vi "Image_Create_Testpattern.vi"(7 "Pattern":enum16{"24 Color Checker", "Customized Pure"}(ring), 8 "error in (no error)":errorcluster, 9 "Pure Color Pattern Parameters":cluster{"R":u8, "G":u8, "B":u8}={"R"=255, "G"=255, "B"=255}, 10 "Image Configuration":T1={"Width"=1920, "Height"=1080}) -> (0 "error out":errorcluster, 1 "Image":T2(plugin-control), 2 "Image Configuration Out":T1={"Width"=1920, "Height"=1080}, 3 "RGB U8":u8[](array[numeric]))   [LabVIEW 2020]
uses:
  ctl/Image_Configuration.ctl
  <vilib>/vision/Image Controls.llb/IMAQ Image.ctl
  <vilib>/vision/NI_Vision_Development_Module.lvlib
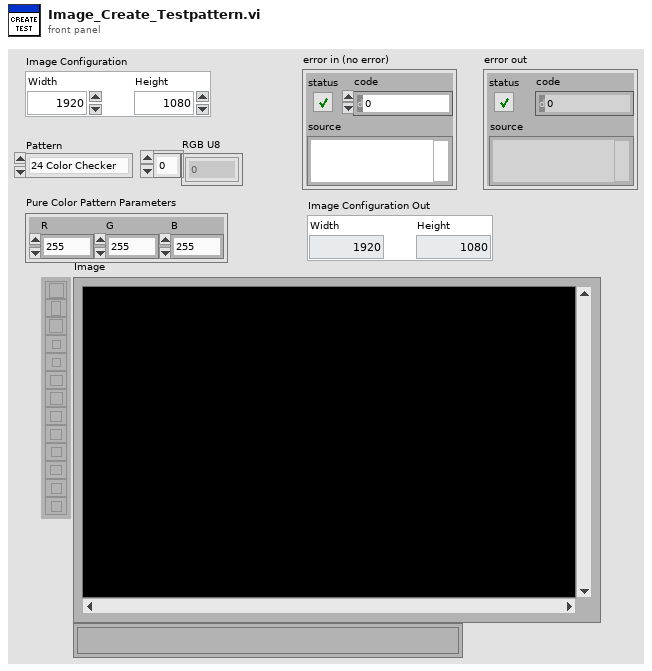
[diagram p1: front panel]
types:
  T1 = typedef "Image_Configuration.ctl" = cluster{"Width":i32, "Height":i32}
  T2 = typedef "IMAQ Image.ctl" = refnum<image>
  T3 = typedef "Image Type" = u32
  T4 = cluster{"Red (or Hue) value":u8, "Green (or Sat) value":u8, "Blue (or Light or Val) value":u8}[]
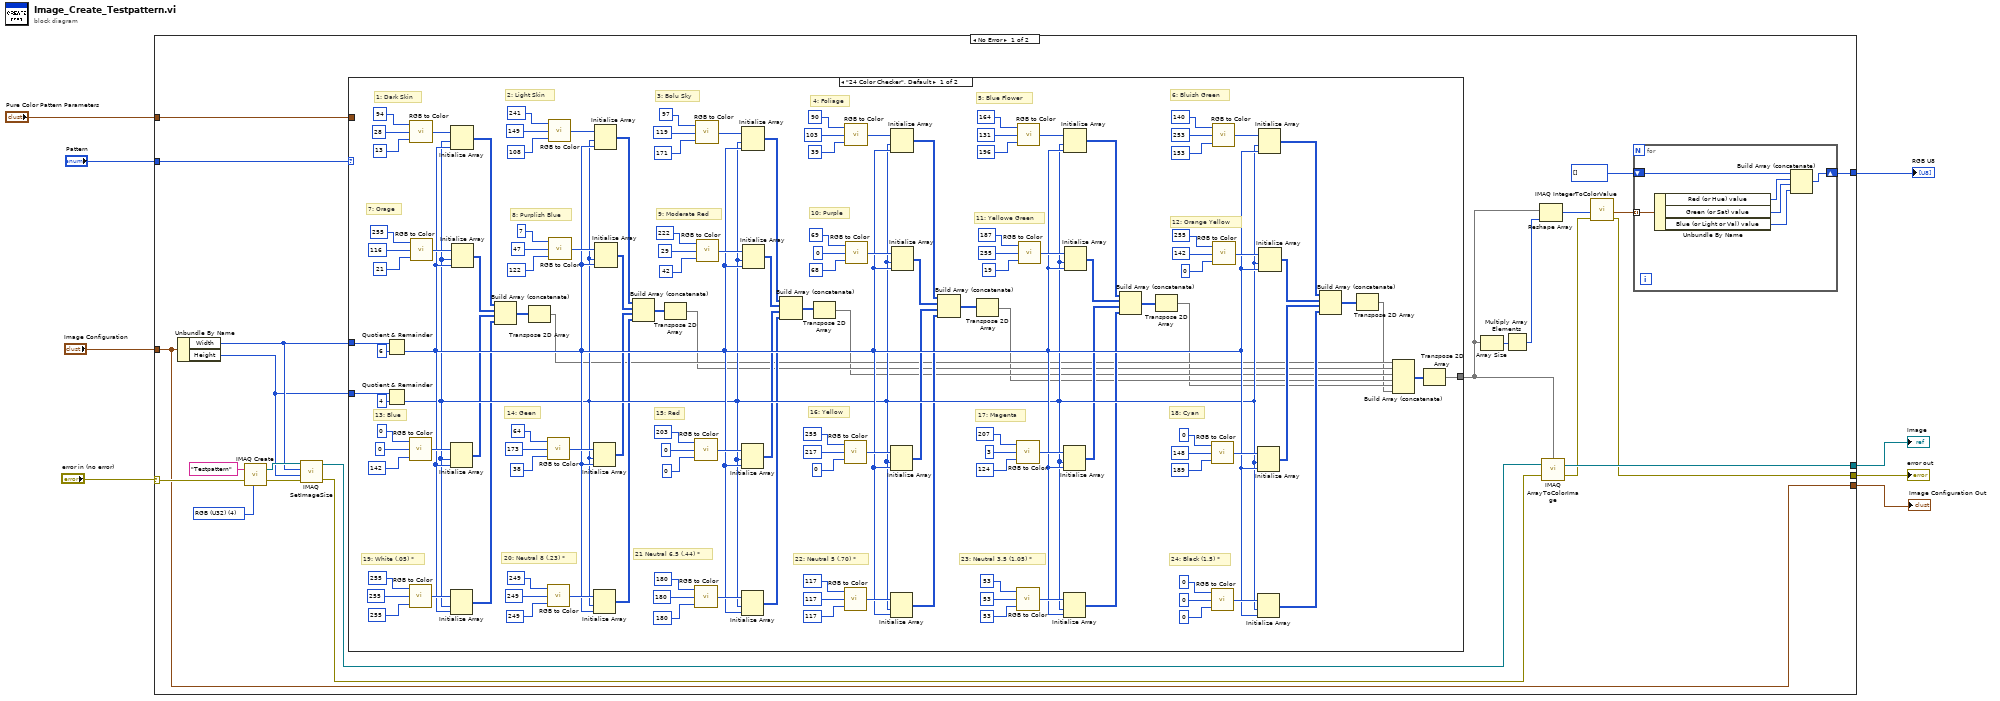
[diagram p0: block diagram]
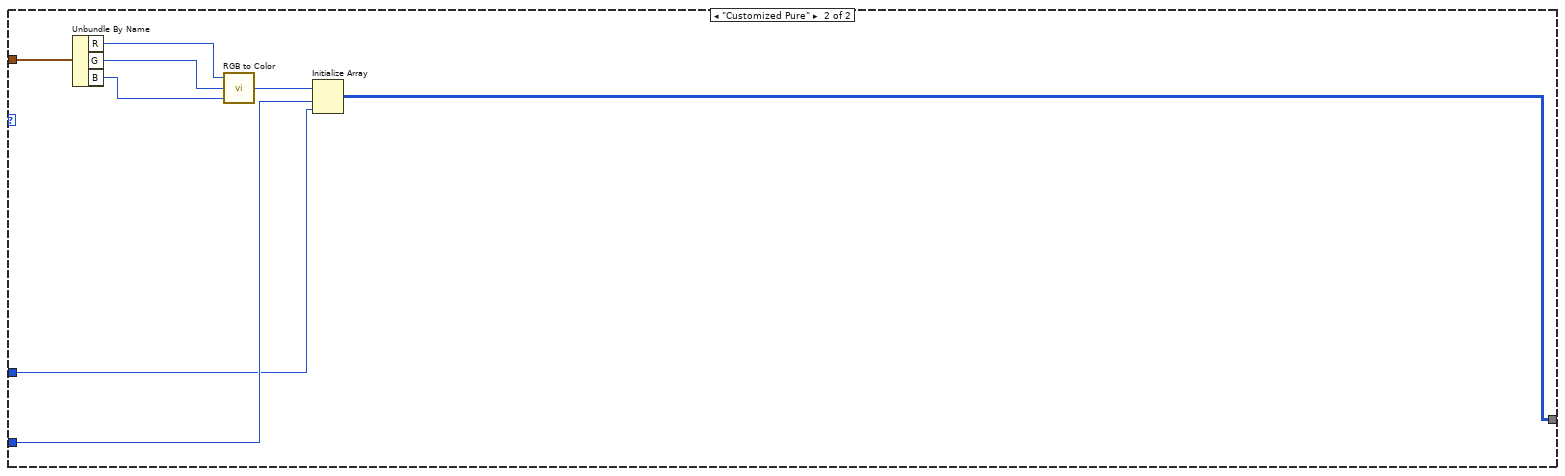
[diagram p2: hidden frame]
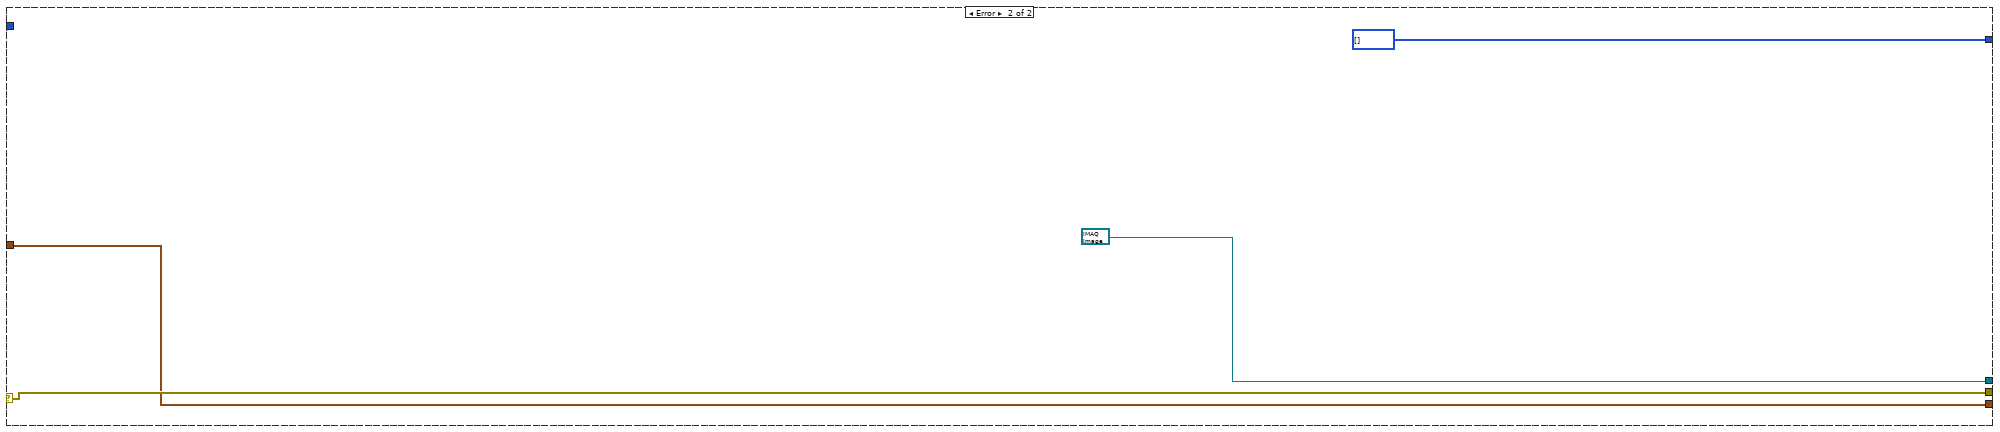
[diagram p3: hidden frame]
diagram:
  n1 = case shown="No Error" "error in (no error)" {
    selector: "error in (no error)" -> [w27 w187]
    tunnel: "Image Configuration" -> [w10 w185]
    tunnel: [w23 T2 refnum ("Image Out")] -> w6
    tunnel: [w14 w187] -> w5
    tunnel: [w15 u8[] []] -> w4
    tunnel: "Pattern" -> [w13 _]
    tunnel: [w10 w185] -> w2
    tunnel: "Pure Color Pattern Parameters" -> [w9 _]
    frame No Error {
      w30 = T3 4 items=["Grayscale (U8)", "Grayscale (I16)", "Grayscale (SGL)", "Complex (CSG)", "RGB (U32)", "HSL (U32)", "RGB (U64)", "Grayscale (U16)"] ("Image Type")
      n2 = Unbundle By Name(w10) -> ("Width"=w25:i32, "Height"=w24:i32)
      n3 = call "IMAQ Create"("Image Name"="Testpattern", "Image Type"=w30, "error in (no error)"=w27) -> ("New Image"=w28:T2, "error out"=w29:errorcluster)  [unwired: 2 in]
      n4 = call "IMAQ SetImageSize"("error in (no error)"=w29, "Y Resolution"=w24, "X Resolution"=w25, "Image"=w28) -> ("error out"=w11:errorcluster, "Image Out"=w12:T2)  [unwired: 1 in]
      n5 = case shown="\"24 Color Checker\", Default" w13 {
        tunnel: w25 -> [w167 w172]
        tunnel: w24 -> [w165 w173]
        tunnel: [w31 w171] -> w20
        tunnel: w9 -> [_ w177]
        frame "24 Color Checker", Default {
          # "24: Black (1.5) *"
          # "23: Neutral 3.5 (1.05) *"
          # "22: Neutral 5 (.70) *"
          # "21 Neutral 6.5 (.44) *"
          # "20: Neutral 8 (.23) *"
          # "19: White (.05) *"
          # "18: Cyan"
          # "17: Magenta"
          # "16: Yellow"
          # "15: Red"
          # "14: Geen"
          # "13: Blue"
          # "12: Orange Yellow"
          # "11: Yellowe Green"
          # "10: Purple"
          # "9: Moderate Red"
          # "8: Purplish Blue"
          # "7: Orage"
          # "6: Bluish Green"
          # "5: Blue Flower"
          # "4: Foliage"
          # "3: Bolu Sky"
          # "2: Light Skin"
          # "1: Dark Skin"
          n6 = Quotient & Remainder(x=w167, y=6) -> (floor(x/y)=w70:i32)  [unwired: 1 out]
          n7 = Quotient & Remainder(x=w165, y=4) -> (floor(x/y)=w69:i32)  [unwired: 1 out]
          n8 = call <vilib>:"RGB to Color.vi"("B"=u8 142, "G"=u8 0, "R"=u8 0) -> ("Color"=w116:u32)
          n9 = call <vilib>:"RGB to Color.vi"("B"=u8 255, "G"=u8 255, "R"=u8 255) -> ("Color"=w92:u32)
          n10 = call <vilib>:"RGB to Color.vi"("B"=u8 13, "G"=u8 28, "R"=u8 94) -> ("Color"=w168:u32)
          n11 = call <vilib>:"RGB to Color.vi"("B"=u8 21, "G"=u8 116, "R"=u8 255) -> ("Color"=w140:u32)
          n12 = Initialize Array(w116, w69, w70) -> (w66:u32[][])
          n13 = Initialize Array(w92, w69, w70) -> (w65:u32[][])
          n14 = Initialize Array(w168, w69, w70) -> (w68:u32[][])
          n15 = Initialize Array(w140, w69, w70) -> (w67:u32[][])
          n16 = Build Array (concatenate)(w68, w67, w66, w65) -> (w44:u32[][])
          n17 = Transpose 2D Array(2D array=w44) -> (transposed array=w38:u32[][])
          n18 = call <vilib>:"RGB to Color.vi"("B"=u8 38, "G"=u8 173, "R"=u8 64) -> ("Color"=w112:u32)
          n19 = call <vilib>:"RGB to Color.vi"("B"=u8 249, "G"=u8 249, "R"=u8 249) -> ("Color"=w88:u32)
          n20 = call <vilib>:"RGB to Color.vi"("B"=u8 108, "G"=u8 149, "R"=u8 241) -> ("Color"=w160:u32)
          n21 = call <vilib>:"RGB to Color.vi"("B"=u8 122, "G"=u8 47, "R"=u8 7) -> ("Color"=w136:u32)
          n22 = Initialize Array(w112, w69, w70) -> (w62:u32[][])
          n23 = Initialize Array(w88, w69, w70) -> (w61:u32[][])
          n24 = Initialize Array(w160, w69, w70) -> (w64:u32[][])
          n25 = Initialize Array(w136, w69, w70) -> (w63:u32[][])
          n26 = Build Array (concatenate)(w64, w63, w62, w61) -> (w43:u32[][])
          n27 = Transpose 2D Array(2D array=w43) -> (transposed array=w37:u32[][])
          n28 = call <vilib>:"RGB to Color.vi"("B"=u8 0, "G"=u8 0, "R"=u8 203) -> ("Color"=w108:u32)
          n29 = call <vilib>:"RGB to Color.vi"("B"=u8 180, "G"=u8 180, "R"=u8 180) -> ("Color"=w84:u32)
          n30 = call <vilib>:"RGB to Color.vi"("B"=u8 171, "G"=u8 119, "R"=u8 97) -> ("Color"=w156:u32)
          n31 = call <vilib>:"RGB to Color.vi"("B"=u8 42, "G"=u8 29, "R"=u8 222) -> ("Color"=w132:u32)
          n32 = Initialize Array(w108, w69, w70) -> (w58:u32[][])
          n33 = Initialize Array(w84, w69, w70) -> (w57:u32[][])
          n34 = Initialize Array(w156, w69, w70) -> (w60:u32[][])
          n35 = Initialize Array(w132, w69, w70) -> (w59:u32[][])
          n36 = Build Array (concatenate)(w60, w59, w58, w57) -> (w42:u32[][])
          n37 = Transpose 2D Array(2D array=w42) -> (transposed array=w36:u32[][])
          n38 = call <vilib>:"RGB to Color.vi"("B"=u8 0, "G"=u8 217, "R"=u8 255) -> ("Color"=w107:u32)
          n39 = call <vilib>:"RGB to Color.vi"("B"=u8 117, "G"=u8 117, "R"=u8 117) -> ("Color"=w83:u32)
          n40 = call <vilib>:"RGB to Color.vi"("B"=u8 39, "G"=u8 103, "R"=u8 90) -> ("Color"=w155:u32)
          n41 = call <vilib>:"RGB to Color.vi"("B"=u8 68, "G"=u8 0, "R"=u8 69) -> ("Color"=w131:u32)
          n42 = Initialize Array(w107, w69, w70) -> (w54:u32[][])
          n43 = Initialize Array(w83, w69, w70) -> (w53:u32[][])
          n44 = Initialize Array(w155, w69, w70) -> (w56:u32[][])
          n45 = Initialize Array(w131, w69, w70) -> (w55:u32[][])
          n46 = Build Array (concatenate)(w56, w55, w54, w53) -> (w41:u32[][])
          n47 = Transpose 2D Array(2D array=w41) -> (transposed array=w35:u32[][])
          n48 = call <vilib>:"RGB to Color.vi"("B"=u8 124, "G"=u8 3, "R"=u8 207) -> ("Color"=w102:u32)
          n49 = call <vilib>:"RGB to Color.vi"("B"=u8 53, "G"=u8 53, "R"=u8 53) -> ("Color"=w78:u32)
          n50 = call <vilib>:"RGB to Color.vi"("B"=u8 196, "G"=u8 131, "R"=u8 164) -> ("Color"=w150:u32)
          n51 = call <vilib>:"RGB to Color.vi"("B"=u8 19, "G"=u8 255, "R"=u8 187) -> ("Color"=w126:u32)
          n52 = Initialize Array(w102, w69, w70) -> (w50:u32[][])
          n53 = Initialize Array(w78, w69, w70) -> (w49:u32[][])
          n54 = Initialize Array(w150, w69, w70) -> (w52:u32[][])
          n55 = Initialize Array(w126, w69, w70) -> (w51:u32[][])
          n56 = Build Array (concatenate)(w52, w51, w50, w49) -> (w40:u32[][])
          n57 = Transpose 2D Array(2D array=w40) -> (transposed array=w34:u32[][])
          n58 = call <vilib>:"RGB to Color.vi"("B"=u8 189, "G"=u8 148, "R"=u8 0) -> ("Color"=w98:u32)
          n59 = call <vilib>:"RGB to Color.vi"("B"=u8 0, "G"=u8 0, "R"=u8 0) -> ("Color"=w74:u32)
          n60 = call <vilib>:"RGB to Color.vi"("B"=u8 153, "G"=u8 253, "R"=u8 140) -> ("Color"=w146:u32)
          n61 = call <vilib>:"RGB to Color.vi"("B"=u8 0, "G"=u8 142, "R"=u8 255) -> ("Color"=w122:u32)
          n62 = Initialize Array(w98, w69, w70) -> (w46:u32[][])
          n63 = Initialize Array(w74, w69, w70) -> (w45:u32[][])
          n64 = Initialize Array(w146, w69, w70) -> (w48:u32[][])
          n65 = Initialize Array(w122, w69, w70) -> (w47:u32[][])
          n66 = Build Array (concatenate)(w48, w47, w46, w45) -> (w39:u32[][])
          n67 = Transpose 2D Array(2D array=w39) -> (transposed array=w33:u32[][])
          n68 = Build Array (concatenate)(w38, w37, w36, w35, w34, w33) -> (w32:u32[][])
          n69 = Transpose 2D Array(2D array=w32) -> (transposed array=w31:u32[][])
        }
        frame "Customized Pure" {
          n70 = Unbundle By Name(w177) -> ("R"=w176:u8, "G"=w175:u8, "B"=w174:u8)
          n71 = call <vilib>:"RGB to Color.vi"("B"=w174, "G"=w175, "R"=w176) -> ("Color"=w178:u32)
          n72 = Initialize Array(w178, w173, w172) -> (w171:u32[][])
        }
      }
      n73 = Array Size(array=w20) -> (size(s)=w22:i32[])
      n74 = Multiply Array Elements(1:w22) -> (0:w21:i32)
      n75 = Reshape Array(w20, w21) -> (w19:u32[])
      n76 = call "IMAQ ArrayToColorImage"("Image Pixels (U32)"=w20, "Image"=w12, "error in (no error)"=w11) -> ("Image Out"=w23:T2, "error out"=w18:errorcluster)  [unwired: 2 in]
      n77 = call "IMAQ IntegerToColorValue"("error in (no error)"=w18, "1D U32 array"=w19) -> ("1D Color value array"=w17:T4, "error out"=w14:errorcluster)  [unwired: 3 in, 2 out]
      n78 = for {
        tunnel: w17 -> [w184] mode=indexing
        shift-right: [w179] -> w15
        shift-left: u8[] [] -> [w183]
        n79 = Unbundle By Name(w184) -> ("Red (or Hue) value"=w182:u8, "Green (or Sat) value"=w181:u8, "Blue (or Light or Val) value"=w180:u8)
        n80 = Build Array (concatenate)(w183, w182, w181, w180) -> (w179:u8[])
      }
    }
    frame Error {
    }
  }
  "error out" <- w5
  "Image" <- w6
  "RGB U8" <- w4
  "Image Configuration Out" <- w2
